vi "FXP_K_times_X_singleAxis.vi"(8 "NS + 1":u8=9, 11 "x_vec":T1=[0.0, 0.0, 0.0, 0.0, 0.0, 0.0, 0.0, 0.0, 0.0, 0.0, 0.0, 0.0, 0.0, 0.0, 0.0, 0.0, 0.0, 0.0, 0.0, 0.0, 0.0, 0.0, 0.0, 0.0, 0.0]) -> (2 "del u_x":fxp<+/-,32,16>)   [LabVIEW 2017]
doc: "Given an input array X and a reference to a memory item, comput the dot product,\neg K.*X. X can be a vector up to length = 9.\n\nND is the size of the vectors.\n\n\nTHIS VI IS DIFFERENT FROM \"SGL_K2_times_xd\" by different sizes allowed."
uses:
  typeDefs/x_vec_type.ctl
  <vilib>/Platform/TimedLoop/XDataNode/timing_clust.ctl
  <vilib>/Platform/TimedLoop/XDataNode/nitl_modes.ctl
  <vilib>/Platform/TimedLoop/XDataNode/wakeup.ctl
  typeDefs/Kz_bram.ctl
  <vilib>/rvi/IPIntegrationNode/IPINode_Typedef/niFpgaIPINodeSupportedFamilies.ctl
  <vilib>/rvi/Emulation/niFpgaSctlEmulationGetInTimedLoop.vi
  <vilib>/rvi/Emulation/niFpgaEmulationReportErrorSimple.vi
  <vilib>/rvi/Emulation/niFpgaGetClockAttributes.vi
  <vilib>/rvi/Emulation/niFpgaCriticalErrorInLSC.vi
  <vilib>/rvi/DataTransferAndStorage/Container/Common/niFpgaContainerExecOnDevCompGetState.vi
  <vilib>/rvi/Emulation/niFpgaEmulationIsFPGAContextNoSignature.vi
  <vilib>/rvi/DataTransferAndStorage/Container/Common/niFpgaContainerGetUniqueNameForEmu.vi
  <vilib>/rvi/Emulation/niFpgaProcessEmulError.vi
  <vilib>/rvi/errors/nirviReportUnexpectedCaseInternalError (U32).vi
  <vilib>/rvi/Memory/Memory_Emulation/niFpgaMemoryEmulationCacheClearOnFirstRun.vi
  <vilib>/rvi/Memory/Memory_Emulation/nirvimemoryEmulationManagerCache_MakeExclusive.vi
  <vilib>/rvi/Memory/Memory_Emulation/niFpgaMemoryEmulationValidateCache.vi
  <vilib>/rvi/Memory/Memory_Emulation/nirvimemoryEmulationManagerCache_InsertValue.vi
  <vilib>/Utility/error.llb/Clear Errors.vi
  <vilib>/rvi/Memory/Memory_Emulation/nirvimemoryEmulationManagerCache_ReleaseExclusive.vi
  <vilib>/rvi/Memory/Memory_Emulation/nirvimemoryEmulationManagerCache_GetValue.vi
  <vilib>/rvi/Memory/Memory_Emulation/nirvimemoryEmulationManagerCache_SetValue.vi
  <vilib>/rvi/Emulation/niFpgaSctlEmulationResourceMgr.vi
  <vilib>/rvi/IPIntegrationNode/IPINode_Utilities/niFpgaIPINodeSimCore.vi
  <vilib>/Platform/TimedLoop/XDataNode/XDataNode.xnode
  <vilib>/rvi/DataTransferAndStorage/Container/XNode/niFpgaContainer.xnode
  <vilib>/rvi/Memory/Memory_Emulation/niFpgaMemoryEmulationRefIn.vi
  <vilib>/rvi/XilinxIP/XIPIN_XNode/niFpgaXIPIN.xnode
  dspAccumulators/MAC1/Multiply_Accumulator_D8DE52605E734182ABB00CFADECE4F1B.dll
  <vilib>/rvi/IPIntegrationNode/IPINode_Xnode/niFpgaIPINode.xnode
  <vilib>/Platform/TimedLoop/XDataNode/XDNodeRunTimeDep.lvlib
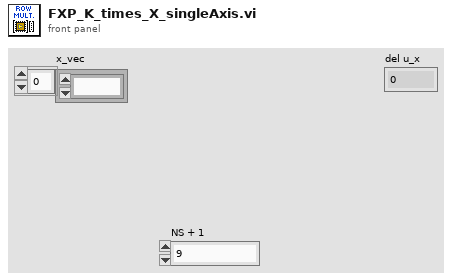
[diagram p1: front panel]
types:
  T1 = typedef "x_vec_type.ctl" = fxp<+/-,32,6>[]
  T2 = typedef "XDNodeRunTimeDep.lvlib/timing_clust.ctl" = cluster{"Expected End [f-1]":u64, "Actual End [f-1]":u64, "Finished Late? [f-1]":bool, "Expected End [i-1]":u64, "Actual End [i-1]":u64, "Finished Late? [i-1]":bool, "Expected Start [i]":u64, "Actual Start [i]":u64, "Expected Start [f]":u64, "Actual Start [f]":u64, "Source Name":string, "Structure Name":string, "Period":i64, "Deadline":i64, "Offset":i64, "Start":i64, "Priority":i32, "Timeout":i32, "Mode":T3, "Wakeup Reason":T4, "Error":errorcluster, "Source Type":string, "Secondary Source Type":string, "Global End Time":u64, "Global Start Time":u64, "Frame Duration":u64, "Iteration Duration":u64, "Assigned CPU":i32, "I/O Scan Engine Mode":u32}
  T3 = typedef "XDNodeRunTimeDep.lvlib/nitl_modes.ctl" = enum32{"No Change", "Process missed periods, maintain original phase", "Discard missed periods, maintain original phase", "Process missed periods, ignore original phase", "Discard missed periods, ignore original phase"}
  T4 = typedef "XDNodeRunTimeDep.lvlib/wakeup.ctl" = enum32{"Normal", "Aborted", "Asynchronous wakeup", "Timing source error", "Timed loop error", "Timeout"}
  T5 = typedef "Kz_bram.ctl" = refnum<k21>
  T6 = typedef "niFpgaIPINodeSupportedFamilies.ctl" = cluster{"unlimited?":bool, "supported targets":string[]}
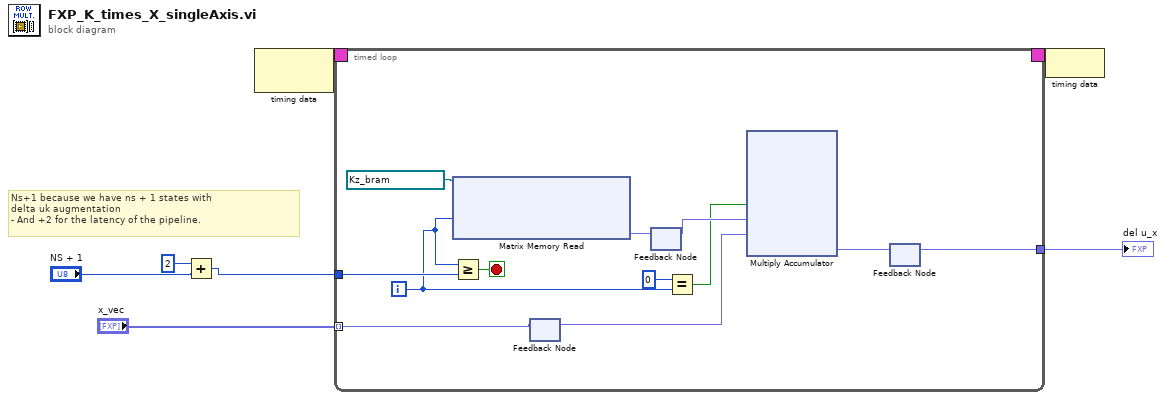
[diagram p0: block diagram]
diagram:
  # "Ns+1 because we have ns + 1 states with \ndelta uk augmentation\n- And +2 for the latency of the pipeline."
  n1 = Add(x=u8 2, y="NS + 1") -> (x+y=w4:u8)
  n2 = node-c288() -> (w7:T2)  [unwired: 1 in]
  n3 = timed-loop {
    timing: w7 -> [_]
    timing-out: [_] -> w6
    tunnel: w4 -> [w18]
    tunnel: [w12] -> w2
    tunnel: "x_vec" -> [w13] mode=indexing
    i -> [w17]
    stop <- w19 stop-if-true
    n4 = xnode "Matrix Memory Read"("Address"=w17, "Memory In"=T5 "K_FXP_row1" ("Memory")) -> ("Data"=w15:fxp<+/-,32,10>)  [unwired: 1 out]
    n5 = Greater Or Equal?(x=w17, y=w18) -> (x >= y?=w19:bool)
    n6 = feedback #1() -> (w14:fxp<+/-,32,6>)  [unwired: 1 in]
    n7 = feedback-in #1(w13) -> ()
    n8 = feedback-in #2(w15) -> ()
    n9 = feedback #2() -> (w10:fxp<+/-,32,10>)  [unwired: 1 in]
    n10 = Equal?(x=0, y=w17) -> (x = y?=w8:bool)
    n11 = xnode ("Multiply Accumulator")("sclr"=w8, "a"=w10, "b"=w14) -> ("s"=w11:fxp<+/-,32,16>)  [unwired: 1 in]
    n12 = feedback #3() -> (w12:fxp<+/-,32,16>)  [unwired: 1 in]
    n13 = feedback-in #3(w11) -> ()
  }
  "del u_x" <- w2
  n14 = node-c288(w6) -> ()
